vi "DebugProg.vi"() -> ()   [LabVIEW 2009]
panel:
  out "ALG output array":T1(array[cluster])
  out "appended path":path
  out "VOC Input varables type":string[](array[string])
  out "VOC Output varables type":string[](array[string])
  out "VOC Input varables names":string[](array[string])
  out "VOC Output varables names":string[](array[string])
  out "VOC Output varables ports":i32[](array[numeric])
  out "VOC Input varables bytes":i32[](array[numeric])
  out "VOC Output varables bytes":i32[](array[numeric])
  out "VOC Input varables ports":i32[](array[numeric])
  out "Array":u8[](array[numeric])
  out "Result Input FOR VOC":u8[](array[numeric])
  out "ALG MSG  PARAM 2":enum16{"void", "byte", "int", "float"}(ring)
  out "CA Output varables names":string[](array[string])
  out "CA Output varables type":string[](array[string])
  out "AY Input varables names":string[](array[string])
  out "AY Input varables type":string[](array[string])
  out "Output ALG Msg Last Iter":string[][](table)
  out "Output VOC Msg Last Iter":string[][](table)
  out "Curr step ALG msg counter":i32
  out "Curr step VOC MSG counter":i32
  in  "Mode":bool
  in  "stop 2":bool
  in  "run":bool
  in  "Tab Control":T2(tab)
  out "Очередь сообщений для АУ":i32(slide)
  in  "send ALG msg":bool
  in  "Параметр сообщения для АУ":string
  in  "Код сообщения для АУ":string(combo)
  out "Очередь сообщений для  ВОУ":i32(slide)
  in  "send voc msg 2":bool
  in  "Параметр сообщения для ВОУ":string
  in  "Код сообщения для ВОУ":string(combo)
  in  "Тип параметра сообщения для АУ":enum16{"void", "byte", "int", "float"}(ring)
  in  "Тип параметра сообщения для ВОУ":enum16{"void", "byte", "int", "float"}(ring)
  out "Выходные глобальные переменные АУ":string[][](table)
  in  "Входные глобальные переменные АУ":string[][](table)
  in  "Значение порта АУ":u8
  in  "Ручное управление портом АУ":bool
  in  "Установить новое значение порта АУ":bool
  in  "ALG Input Ports":i32(listbox) caption="Входные порты АУ"
  out "Выходные глобальные переменные ВОУ":string[][](table)
  in  "Значение порта ВОУ":u8
  in  "Ручное управление портом ВОУ":bool
  in  "Установить новое значение порта ВОУ":bool
  in  "Входные глобальные переменные ВОУ":string[][](table)
  in  "Входные порты ВОУ":i32(listbox)
  in  "Выходные сообщения от АУ на последнем шаге":i32(listbox)
  out "Отладочная информация процессов АУ":string[][](table)
  out "Список выходных сообщений от АУ":string[][](table)
  in  "Выходные сообщения от ВОУ на последнем шаге":i32(listbox)
  out "Список выходных сообщений от ВОУ":string[][](table)
  out "Отладочная информация процессов ВОУ":string[][](table)
  in  "stop":bool
  # "ПОШАГОВЫЙ РЕЖИМ"
  # "НЕПРЕРЫВНЫЙ РЕЖИМ"
  # "Входные сообщения АУ"
  # "Входные сообщения ВОУ"
  # "Порядок создания нового проекта:\n\n1)\tИз папки \"C:\\ProgramData\\ManualComplexData\" Скопируйте папки CA, VOC и файл cfg.xml в директорию проекта. \n2)\tЗакройте программу ручной отладки, если она была у вас открыта.\n3)\tВ папке CA в файле CA.rcs опишите алгоритм управления. Запустите скрипт ManualBuild.\n4)\tВ папке VOC в файле voc.rcs опишите алгоритм управления. Запустите скрипт ManualBuild."
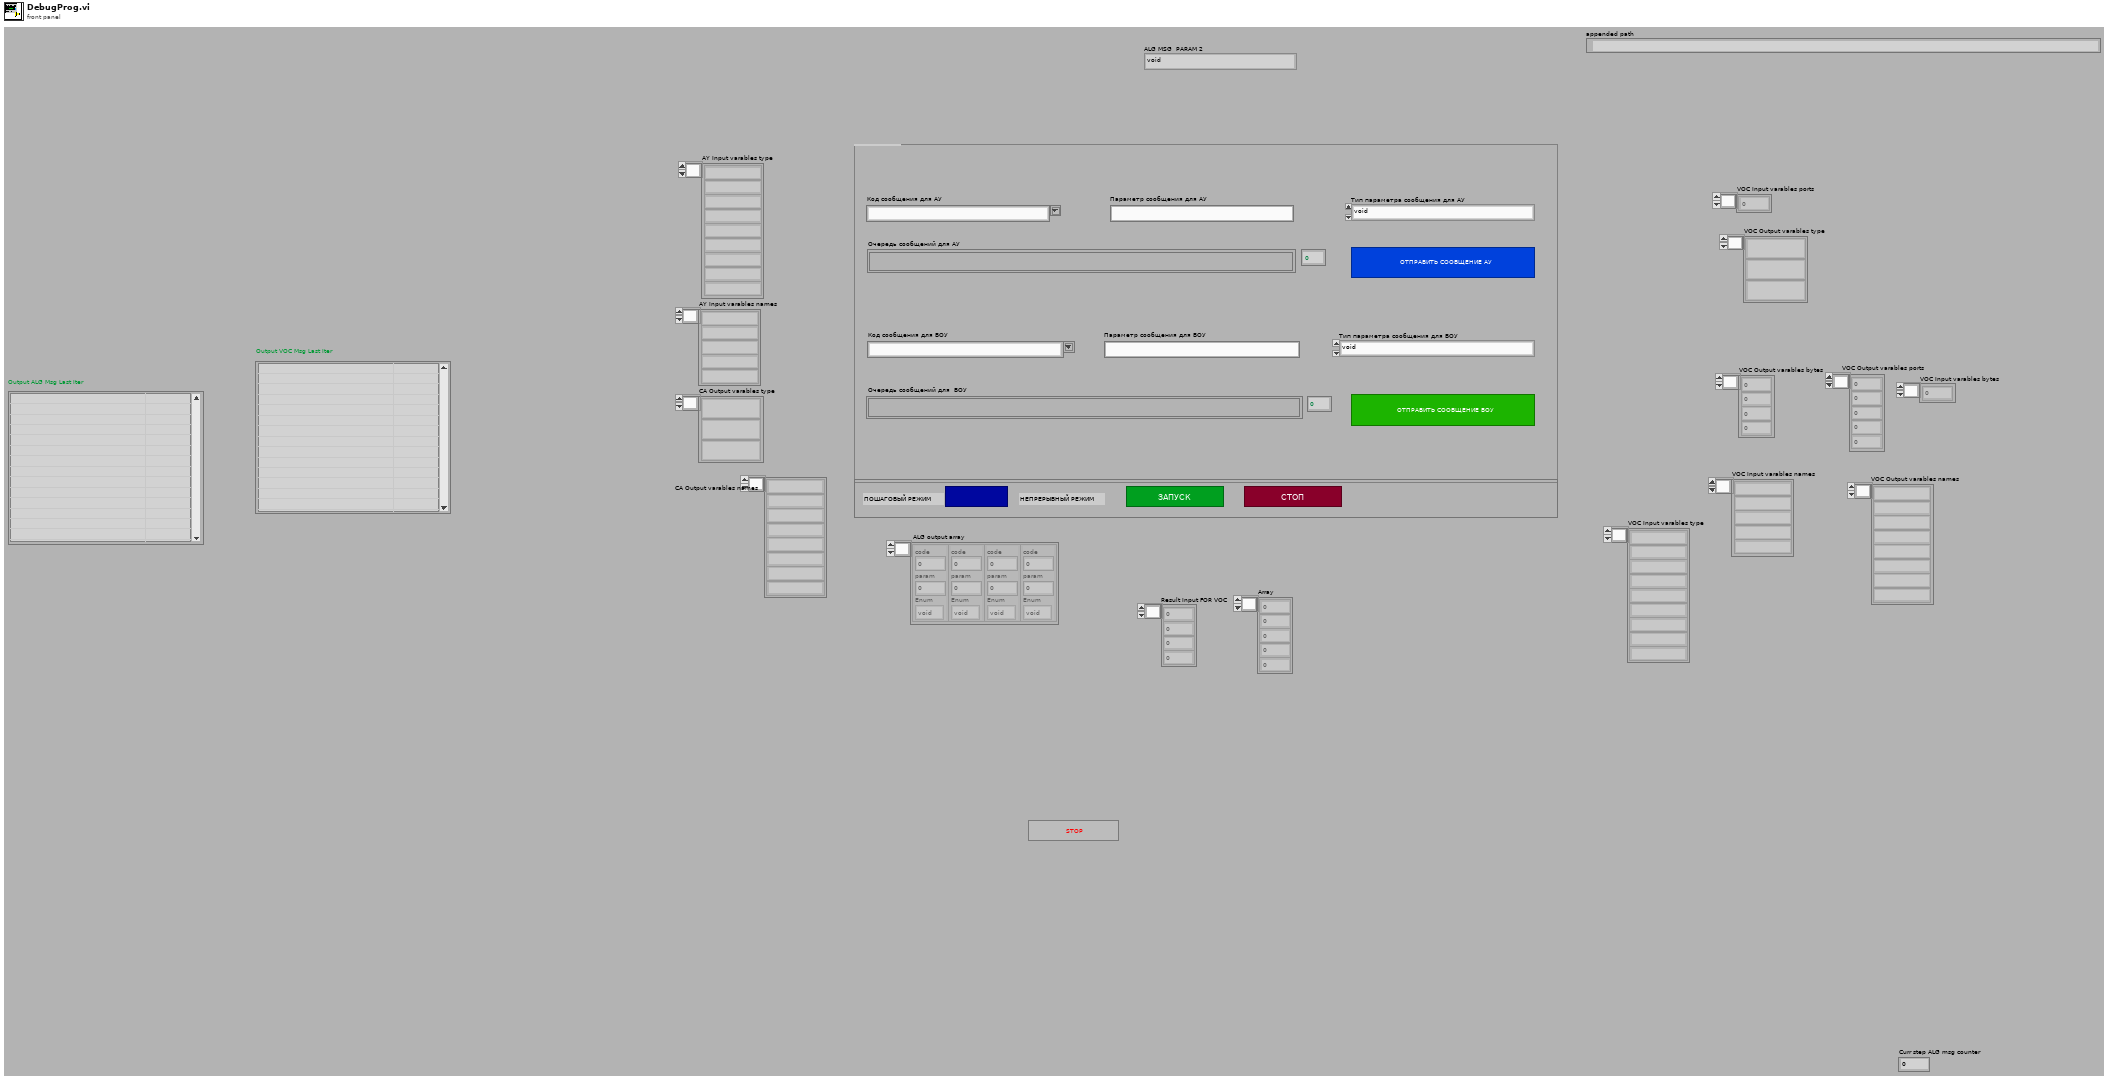
[diagram p1: front panel]
types:
  T1 = cluster{"code":i32, "param":i32, "Enum":enum16{"void", "byte", "int", "float"}}[]
  T2 = enum32{"Генерация входных сообщений АУ и ВОУ", "Переменные АУ", "Переменные ВОУ", "Отладочная информация АУ", "Отладочная информация ВОУ", "Помощь"}
  T3 = enum8{"Enabled", "Disabled", "Disabled and Grayed Out"}
  T4 = cluster{"code":i32, "param":i32, "Enum":enum16{"void", "byte", "int", "float"}}
  T5 = cluster{"trimmed string":string, "trimmed string":string}[]
  T6 = cluster{i32, "Casted Parameter":i32, "Тип параметра сообщения для АУ":enum16{"void", "byte", "int", "float"}}
  T7 = cluster{i32, "Casted Parameter":i32, "Тип параметра сообщения для ВОУ":enum16{"void", "byte", "int", "float"}}
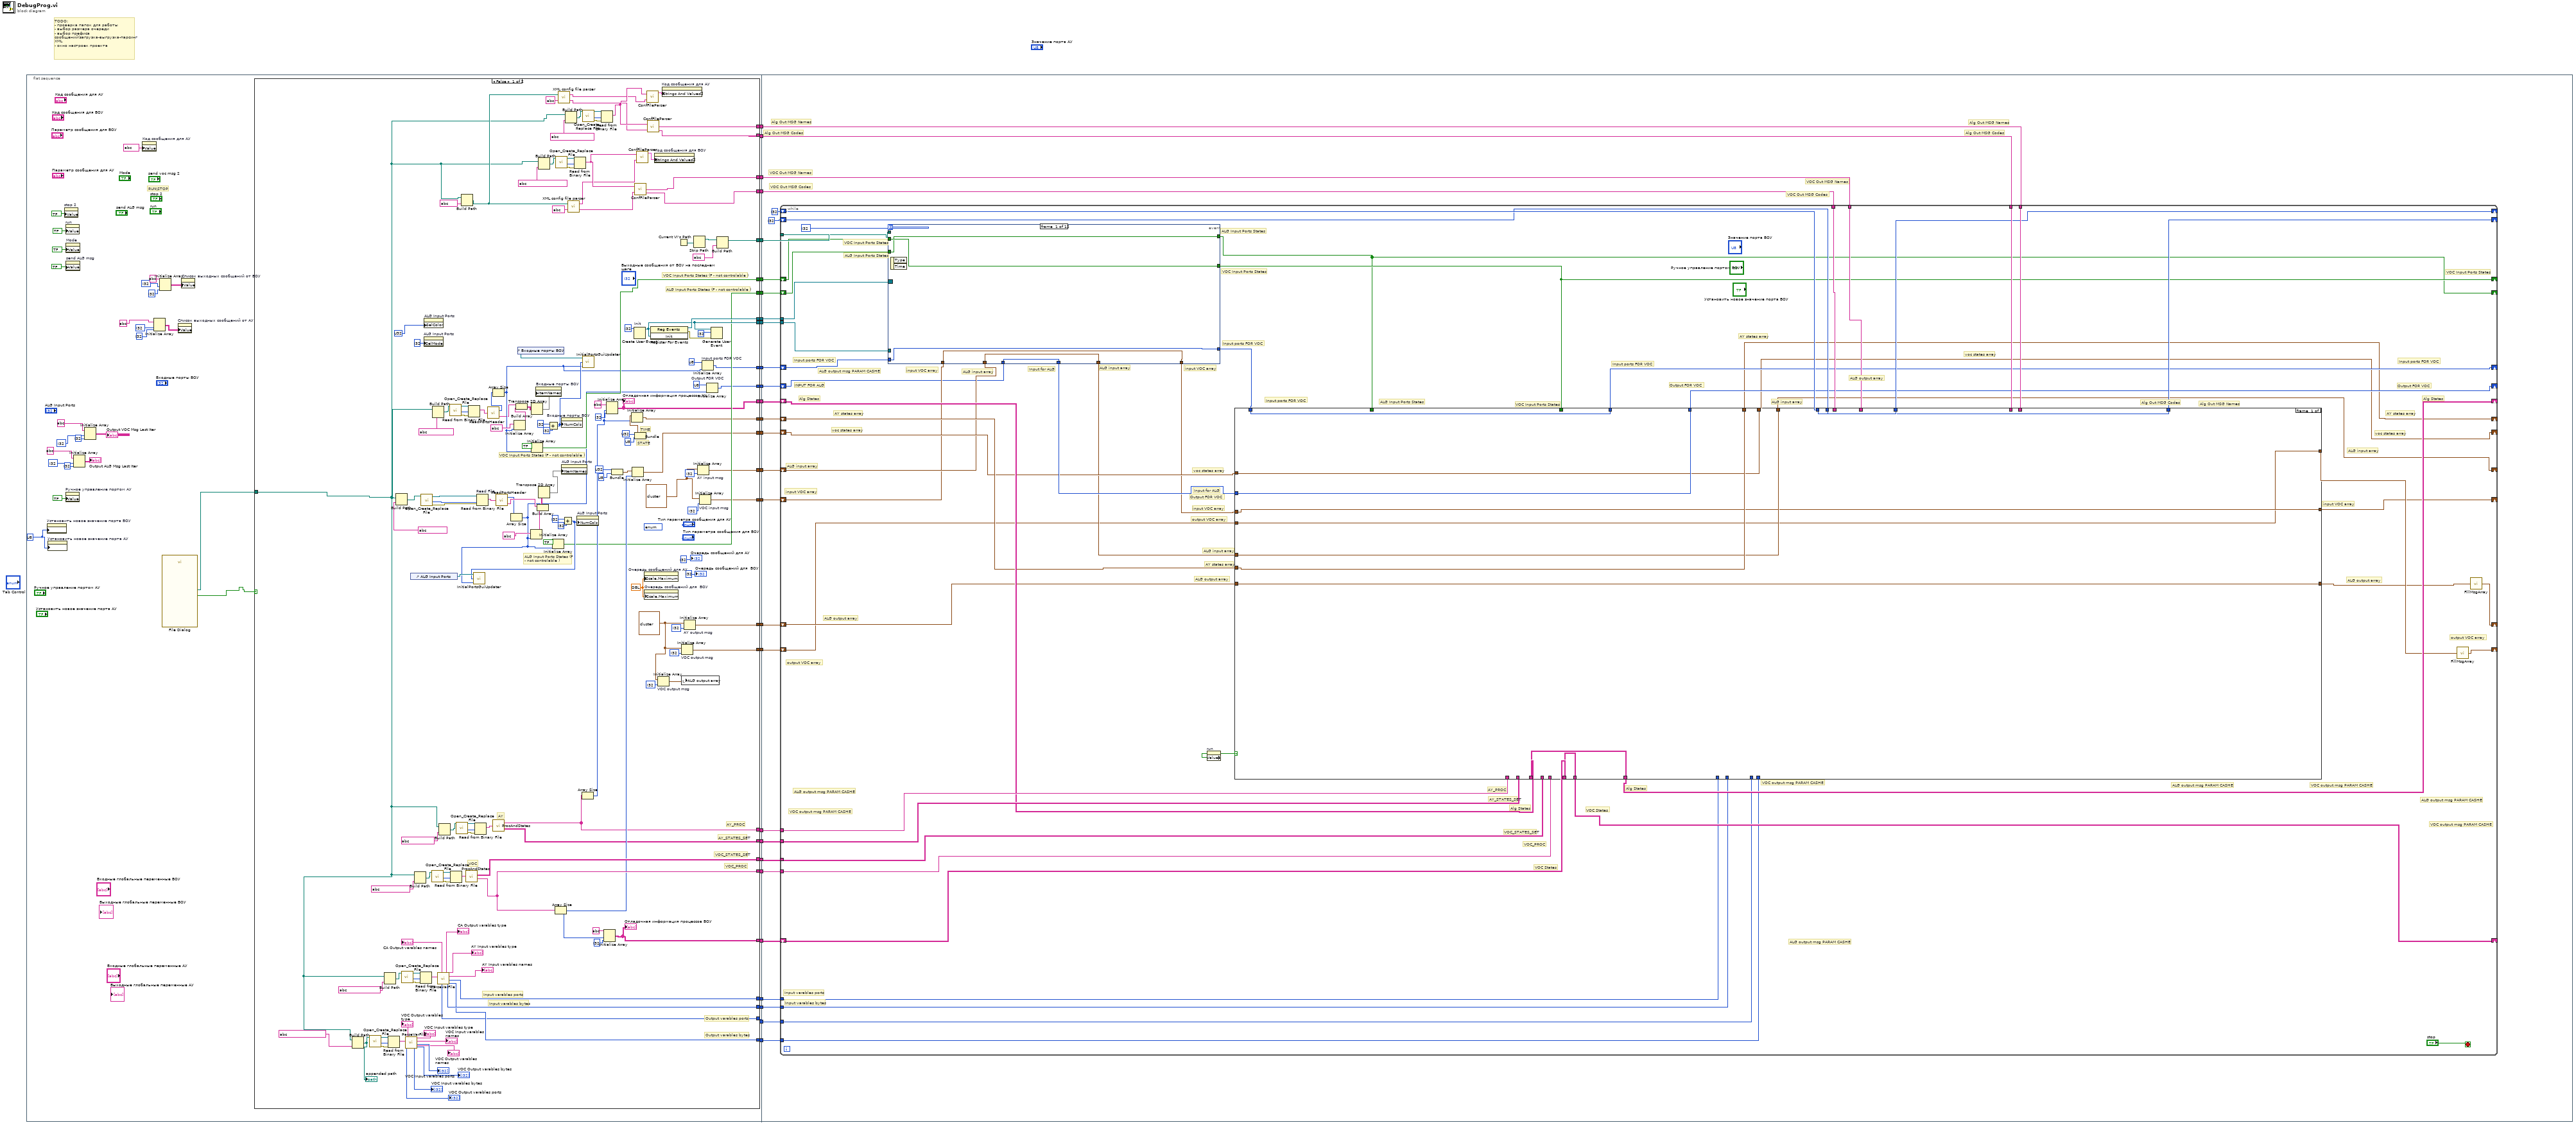
[diagram p0: block diagram]
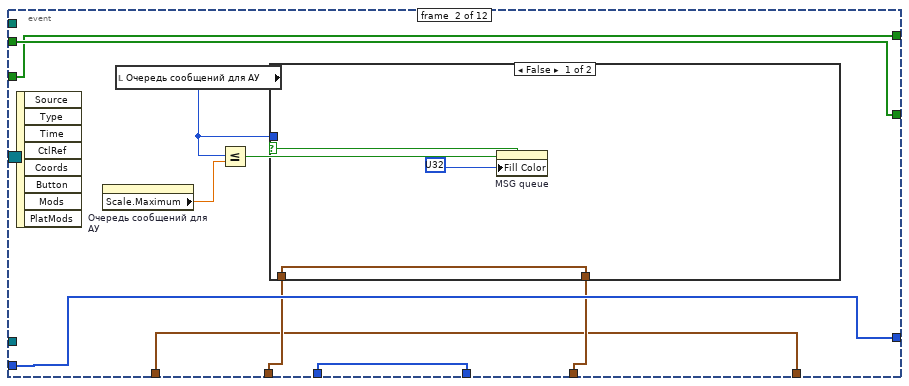
[diagram p3: hidden frame]
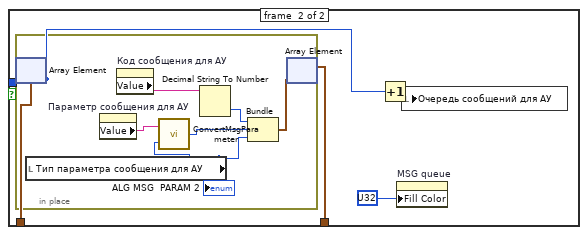
[diagram p4: hidden frame]
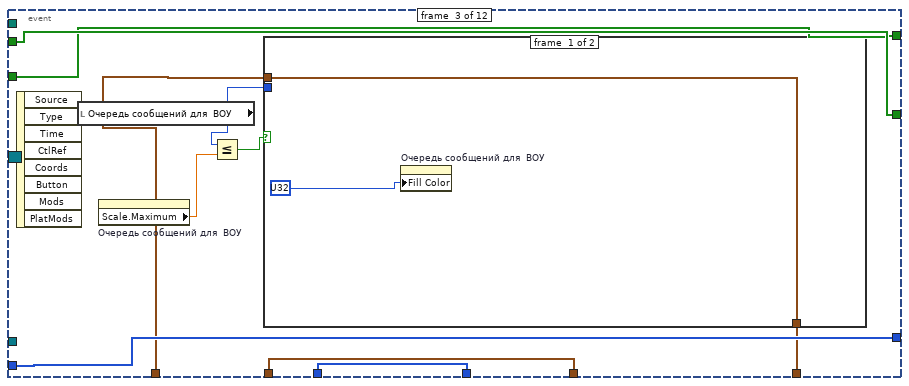
[diagram p5: hidden frame]
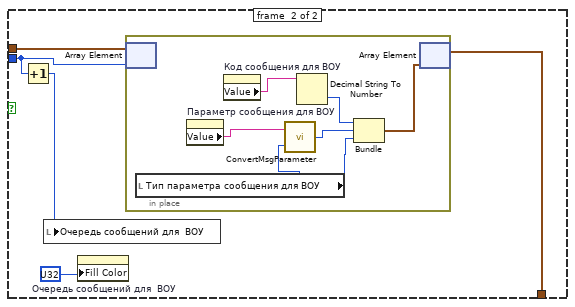
[diagram p6: hidden frame]
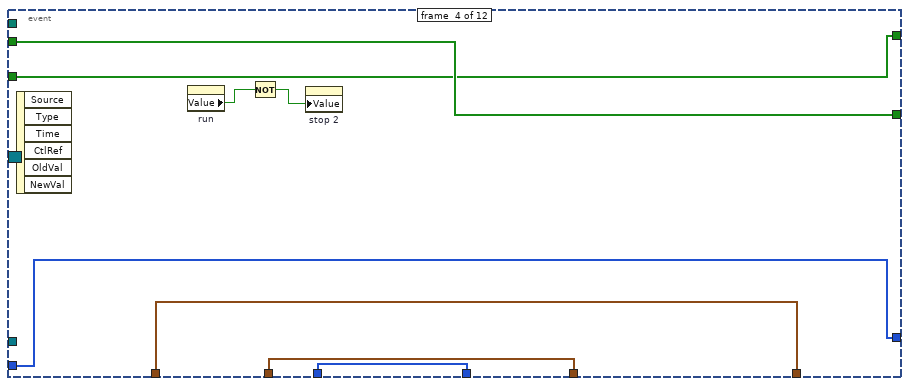
[diagram p7: hidden frame]
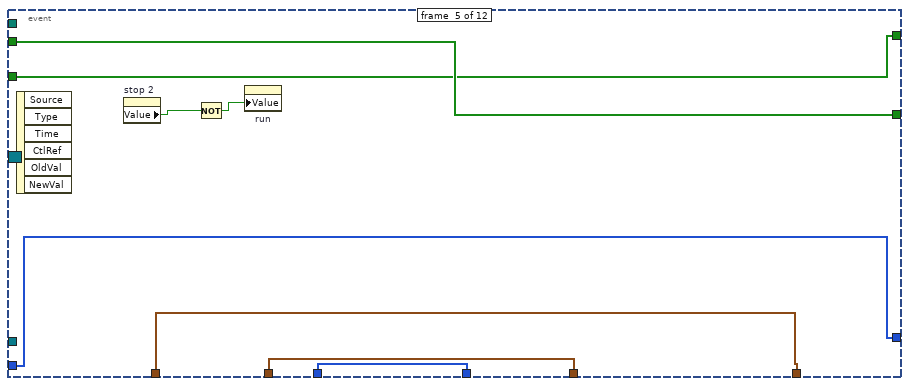
[diagram p8: hidden frame]
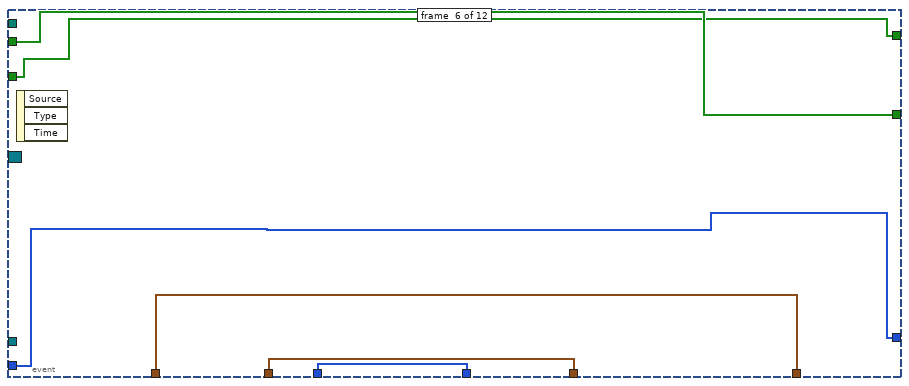
[diagram p9: hidden frame]
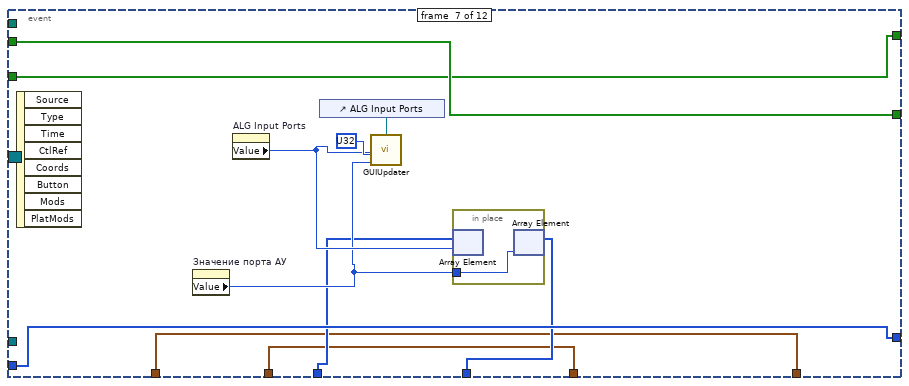
[diagram p10: hidden frame]
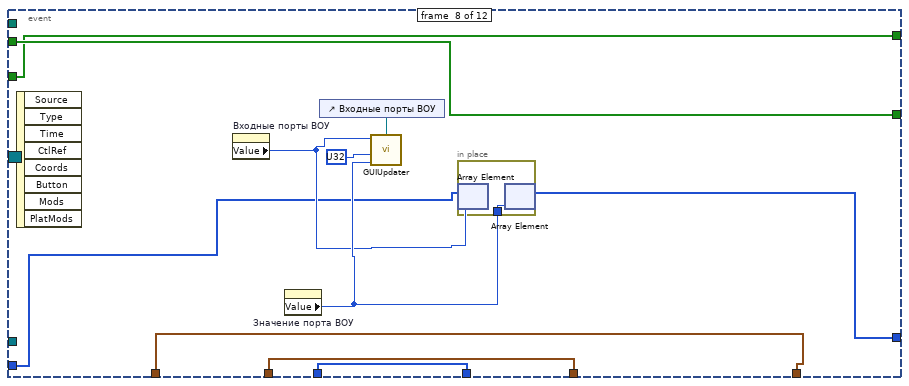
[diagram p11: hidden frame]
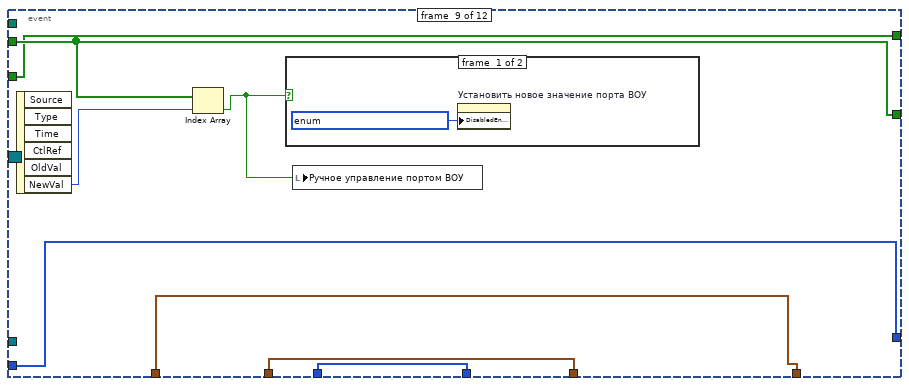
[diagram p12: hidden frame]
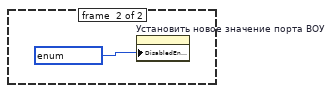
[diagram p13: hidden frame]
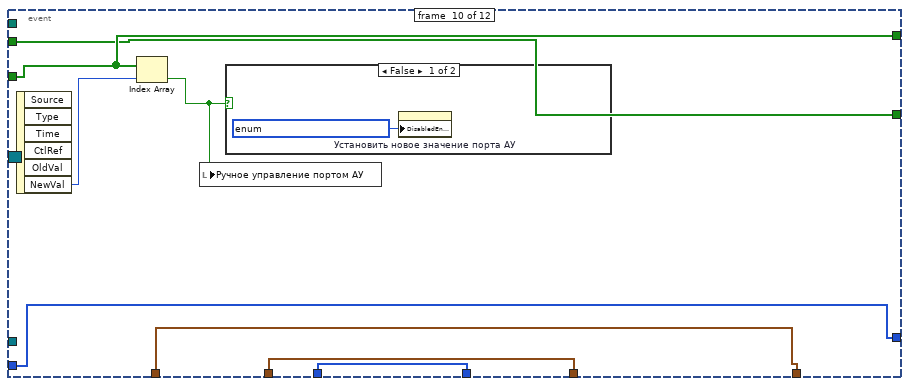
[diagram p14: hidden frame]
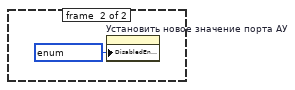
[diagram p15: hidden frame]
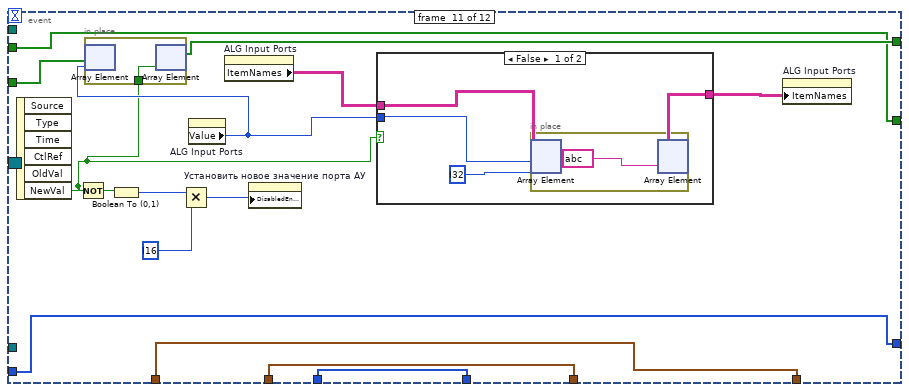
[diagram p16: hidden frame]
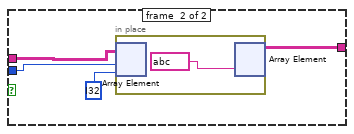
[diagram p17: hidden frame]
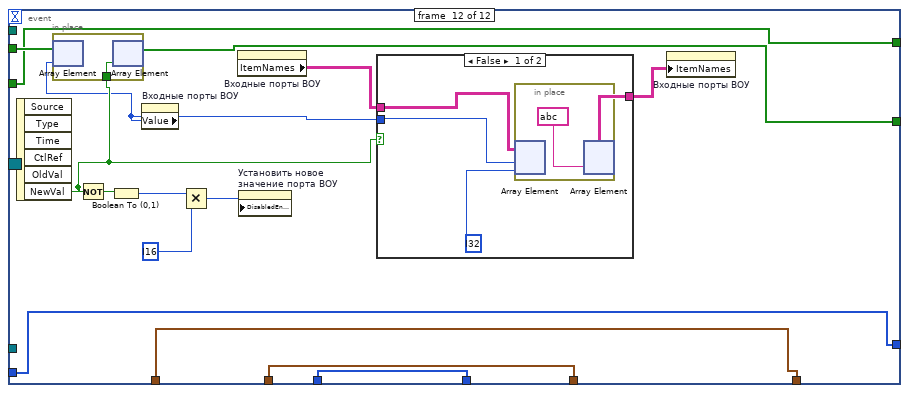
[diagram p18: hidden frame]
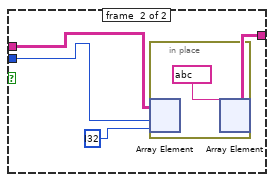
[diagram p19: hidden frame]
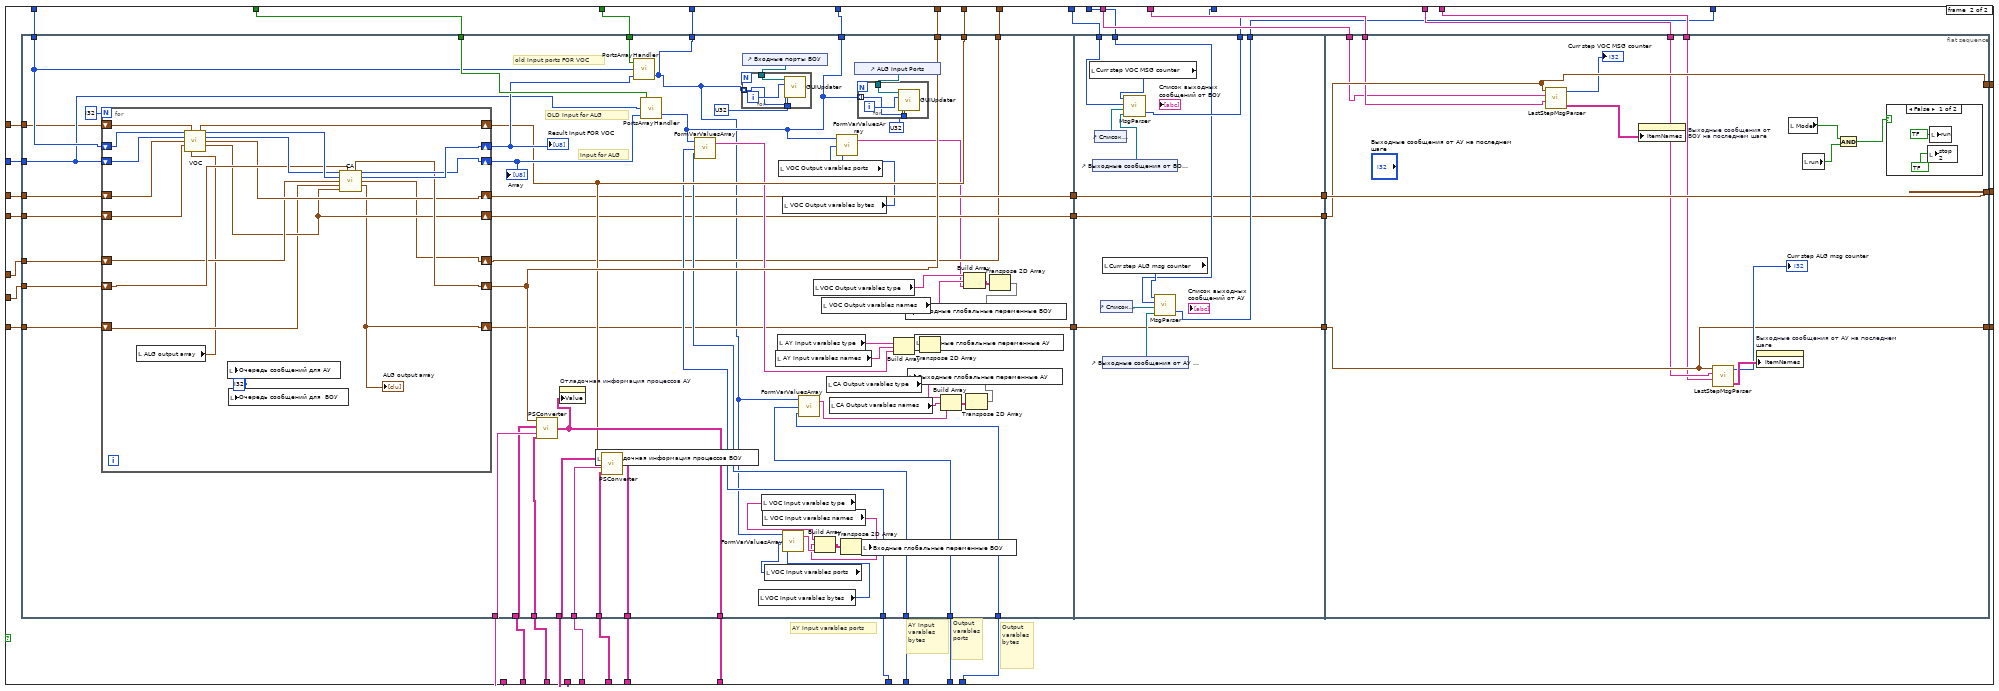
[diagram p20: hidden frame]
diagram:
  # "TODO:\n- проверка папок для работы\n- выбор размера очереди\n- выбор префиса сообщений(загрузка-выгрузка-парсинг XML\n- окно настроек проекта"
  n1 = flat-sequence {
    tunnel: [w74] -> w27
    tunnel: [w72] -> w26
    tunnel: [w73] -> w25
    tunnel: [w71] -> w24
    tunnel: [w70] -> w23
    tunnel: [w69] -> w22
    tunnel: [w68] -> w21
    tunnel: [w47] -> w20
    tunnel: [w46] -> w19
    tunnel: [w58] -> w18
    tunnel: [w61] -> w17
    tunnel: [w45] -> w16
    tunnel: [w44] -> w15
    tunnel: [w43] -> w14
    tunnel: [w42] -> w13
    tunnel: [w41] -> w12
    tunnel: [w40] -> w11
    tunnel: [w39] -> w10
    tunnel: [w38] -> w9
    tunnel: [w37] -> w8
    tunnel: [w36] -> w7
    tunnel: [w35] -> w6
    tunnel: [w34] -> w5
    tunnel: [w31] -> w4
    tunnel: [w33] -> w3
    tunnel: [w30] -> w2
    tunnel: [w32] -> w1
    tunnel: w27 -> [w263]
    tunnel: w26 -> [w262]
    tunnel: w25 -> [w261]
    tunnel: w24 -> [w258]
    tunnel: w23 -> [w257]
    tunnel: w22 -> [w260]
    tunnel: w21 -> [w259]
    tunnel: w20 -> [w255]
    tunnel: w19 -> [w254]
    tunnel: w18 -> [w253]
    tunnel: w17 -> [w252]
    tunnel: w16 -> [w250]
    tunnel: w15 -> [w249]
    tunnel: w14 -> [w248]
    tunnel: w13 -> [w247]
    tunnel: w12 -> [w246]
    tunnel: w11 -> [w245]
    tunnel: w10 -> [w244]
    tunnel: w9 -> [w238]
    tunnel: w8 -> [w237]
    tunnel: w7 -> [w236]
    tunnel: w6 -> [w235]
    tunnel: w5 -> [w243]
    tunnel: w4 -> [w242]
    tunnel: w3 -> [w241]
    tunnel: w2 -> [w240]
    tunnel: w1 -> [w239]
    frame #0 {
      w48 = u8 ? ("Disabled")
      # "RUN\\STOP"
      n2 = property on="Установить новое значение порта ВОУ" class="Bool (strict)"("DisabledEnum"=w48) -> ()  [unwired: 2 in, 2 out]
      n3 = property on="Установить новое значение порта АУ" class="Bool (strict)"("DisabledEnum"=w48) -> ()  [unwired: 2 in, 2 out]
      n4 = property on="stop 2" class="Bool (strict)"("Value"=bool ? ("send msg 3")) -> ()  [unwired: 2 in, 2 out]
      n5 = property on="run" class="Bool (strict)"("Value"=bool ? ("send msg 2")) -> ()  [unwired: 2 in, 2 out]
      n6 = property on="Ручное управление портом АУ" class="Bool (strict)"("Value"=bool ? ("Controlable")) -> ()  [unwired: 2 in, 2 out]
      n7 = property on="Mode" class="Bool (strict)"("Value"=bool ? ("Mode")) -> ()  [unwired: 2 in, 2 out]
      n8 = property on="send ALG msg" class="Bool (strict)"("Value"=bool ? ("send msg")) -> ()  [unwired: 2 in, 2 out]
      n9 = Initialize Array(string ? ("Value"), i32 ? ("dimension size"), i32 ? ("dimension size")) -> (→"Output ALG Msg Last Iter":string[][])
      n10 = Initialize Array(string ? ("Value"), i32 ? ("dimension size"), i32 ? ("dimension size")) -> (→"Output VOC Msg Last Iter":string[][])
      n11 = property on="Код сообщения для АУ" class="CmbBox"("Value"=string ? ("CODE")) -> ()  [unwired: 2 in, 2 out]
      n12 = Initialize Array(string ? ("element"), i32 ? ("dimension size"), i32 ? ("dimension size")) -> (w66:string[][])
      n13 = Initialize Array(string ? ("element"), i32 ? ("dimension size"), i32 ? ("dimension size")) -> (w67:string[][])
      n14 = call "File Dialog"() -> ("selected path"=w29:path, "cancelled"=w28:bool)  [unwired: 12 in, 2 out]
      n15 = property on="Список выходных сообщений от АУ" class="Tbl (strict)"("Value"=w66) -> ()  [unwired: 2 in, 2 out]
      n16 = property on="Список выходных сообщений от ВОУ" class="Tbl (strict)"("Value"=w67) -> ()  [unwired: 2 in, 2 out]
      n17 = case shown="False" w28 {
        tunnel: [w195 _] -> w74
        tunnel: [w191 _] -> w73
        tunnel: [w189 _] -> w72
        tunnel: [w187 _] -> w71
        tunnel: [w186 _] -> w70
        tunnel: [w185 _] -> w69
        tunnel: [w184 _] -> w68
        tunnel: [w178 _] -> w61
        tunnel: [w177 _] -> w58
        tunnel: [w152 _] -> w47
        tunnel: [w151 _] -> w46
        tunnel: [w148 _] -> w45
        tunnel: [w146 _] -> w44
        tunnel: [w143 _] -> w43
        tunnel: [w142 _] -> w42
        tunnel: [w141 _] -> w41
        tunnel: [w140 _] -> w40
        tunnel: [w139 _] -> w39
        tunnel: [w138 _] -> w38
        tunnel: [w137 _] -> w37
        tunnel: [w136 _] -> w36
        tunnel: [w135 _] -> w35
        tunnel: [w134 _] -> w34
        tunnel: [w127 _] -> w33
        tunnel: [w126 _] -> w32
        tunnel: [w119 _] -> w31
        tunnel: [w108 _] -> w30
        tunnel: w29 -> [w83 _]
        frame #0 {
          w107 = dbl ? ("Scale.Range:Maximum")
          (unwired) enum16{"void", "byte", "int", "float"} ? ("Enum")
          w120 = T4 ? ("Cluster")
          w80 = T4 ? ("Cluster")
          w194 = i32 ?  # Init
          # "Output varables bytes"
          # "Output varables ports"
          # "Input varables bytes"
          # "Input varables ports"
          # "VOC Input Ports States (F - not controlable )"
          # "ALG Input Ports States (F - not controlable )"
          # "VOC Input Ports States (F - not controlable )"
          # "ALG Input Ports States (F - not controlable )"
          # "AY"
          # "VOC"
          # "VOC_STATES_SET"
          # "VOC_PROC"
          # "AY_STATES_SET"
          # "AY_PROC"
          # "STATE"
          # "TIME"
          n18 = Build Path(base path=w83, name or relative path=string ?) -> (appended path=w94:path)
          "appended path" <- w94
          n19 = call <vilib>:"Open_Create_Replace File.vi"("file path"=w94) -> ("error out"=w104:errorcluster, "file size (bytes)"=w105:i32, "refnum"=w93:refnum<file>)  [unwired: 7 in, 1 out]
          n20 = Build Path(base path=w83, name or relative path=string ?) -> (appended path=w131:path)
          n21 = Read from Binary File(8:w104, 10:w105, 11:w93) -> (2:w106:string)  [unwired: 3 in, 3 out]
          n22 = Build Path(base path=w83, name or relative path=string ?) -> (appended path=w175:path)
          n23 = call <vilib>:"Open_Create_Replace File.vi"("file path"=w131) -> ("error out"=w133:errorcluster, "file size (bytes)"=w132:i32, "refnum"=w121:refnum<file>)  [unwired: 7 in, 1 out]
          n24 = call "ParseVarFile.vi"("data"=w106) -> ("Output varables bytes"=→"VOC Output varables bytes":i32[], "Output varables names"=→"VOC Output varables names":string[], "Input varables ports"=→"VOC Input varables ports":i32[], "Input varables names"=→"VOC Input varables names":string[], "Output varables type"=→"VOC Output varables type":string[], "Input varables type"=→"VOC Input varables type":string[], "Input varables bytes"=→"VOC Input varables bytes":i32[], "Output varables ports"=→"VOC Output varables ports":i32[])
          n25 = control-ref of="ALG Input Ports"() -> (w157:refnum<vi>)
          n26 = Build Path(base path=w83, name or relative path=string ?) -> (appended path=w214:path)
          n27 = Read from Binary File(8:w133, 10:w132, 11:w121) -> (2:w130:string)  [unwired: 3 in, 3 out]
          n28 = call <vilib>:"Open_Create_Replace File.vi"("file path"=w175) -> ("error out"=w174:errorcluster, "file size (bytes)"=w173:i32, "refnum"=w172:refnum<file>)  [unwired: 7 in, 1 out]
          n29 = property on="ALG Input Ports" class="MCListbox (strict)"("SelMode"=i32 ? ("Selection Mode")) -> ()  [unwired: 2 in, 2 out]
          n30 = property on="ALG Input Ports" class="MCListbox (strict)"("SelColor"=u32 ?) -> ()  [unwired: 2 in, 2 out]
          n31 = call <vilib>:"Open_Create_Replace File.vi"("file path"=w214) -> ("error out"=w213:errorcluster, "file size (bytes)"=w212:i32, "refnum"=w211:refnum<file>)  [unwired: 7 in, 1 out]
          n32 = Build Path(base path=w83, name or relative path=string ?) -> (appended path=w166:path)
          n33 = call "ParseVarFile.vi"("data"=w130) -> ("Output varables bytes"=w126:i32[], "Output varables names"=→"CA Output varables names":string[], "Input varables ports"=w119:i32[], "Input varables names"=→"AY Input varables names":string[], "Output varables type"=→"CA Output varables type":string[], "Input varables type"=→"AY Input varables type":string[], "Input varables bytes"=w127:i32[], "Output varables ports"=w108:i32[])
          n34 = Build Path(base path=w83, name or relative path=string ?) -> (appended path=w208:path)
          n35 = call <vilib>:"Open_Create_Replace File.vi"("file path"=w166) -> ("error out"=w165:errorcluster, "file size (bytes)"=w164:i32, "refnum"=w163:refnum<file>)  [unwired: 7 in, 1 out]
          n36 = Read from Binary File(8:w213, 10:w212, 11:w211) -> (2:w188:string)  [unwired: 3 in, 3 out]
          n37 = call <vilib>:"Open_Create_Replace File.vi"("file path"=w208) -> ("error out"=w207:errorcluster, "file size (bytes)"=w206:i32, "refnum"=w205:refnum<file>)  [unwired: 7 in, 1 out]
          n38 = Build Path(base path=w83, name or relative path=string ?) -> (appended path=w85:path)
          n39 = call "ProcAndStates.vi"("spreadsheet string"=w188) -> ("PROCESSES"=w177:string[], "STATES"=w178:string[][])
          n40 = Read from Binary File(8:w165, 10:w164, 11:w163) -> (2:w118:string)  [unwired: 3 in, 3 out]
          n41 = Read from Binary File(8:w207, 10:w206, 11:w205) -> (2:w216:string)  [unwired: 3 in, 3 out]
          n42 = Read from Binary File "Read File"(8:w174, 10:w173, 11:w172) -> (2:w113:string)  [unwired: 3 in, 3 out]
          n43 = call "ReadPortsHeader.vi"("data"=w118) -> ("Numbers"=w117:i32[], "Names"=w115:string[])
          n44 = Array Size(array=w117) -> (size(s)=w116:i32)
          n45 = call "ProcAndStates.vi"("spreadsheet string"=w216) -> ("PROCESSES"=w152:string[], "STATES"=w151:string[][])
          n46 = call "ReadPortsHeader.vi"("data"=w113) -> ("Numbers"=w110:i32[], "Names"=w112:string[])
          n47 = Array Size(array=w110) -> (size(s)=w109:i32)
          n48 = Initialize Array(string ? ("name or relative path"), w116) -> (w160:string[])
          n49 = Build Array(w115, w160) -> (w159:string[][])
          n50 = control-ref of="Входные порты ВОУ"() -> (w155:refnum<vi>)
          n51 = Initialize Array(string ? ("name or relative path"), w109) -> (w169:string[])
          n52 = Transpose 2D Array(2D array=w159) -> (transposed array=w147:string[][])
          n53 = Initialize Array(bool ? ("Controlable"), w116) -> (w146:bool[])
          n54 = property on="Входные порты ВОУ" class="MCListbox (strict)"("ItemNames"=w147) -> ()  [unwired: 2 in, 2 out]
          n55 = Build Array(w112, w169) -> (w170:string[][])
          n56 = Build Path(base path=w83, name or relative path=string ?) -> (appended path=w229:path)
          n57 = Transpose 2D Array(2D array=w170) -> (transposed array=w168:string[][])
          n58 = Add(x=i32 ?, y=i32 ?) -> (x+y=w154:i32)
          n59 = Initialize Array(bool ? ("Controlable"), w109) -> (w148:bool[])
          n60 = Array Size(array=w177) -> (size(s)=w176:i32)
          n61 = call <vilib>:"Open_Create_Replace File.vi"("file path"=w229) -> ("error out"=w228:errorcluster, "file size (bytes)"=w227:i32, "refnum"=w226:refnum<file>)  [unwired: 7 in, 1 out]
          n62 = call "XML config file parser.vi"("Tag Name"=string ?, "XML File Path"=w85) -> ("Out"=w90:string, "In"=w91:string)
          n63 = property on="Входные порты ВОУ" class="MCListbox (strict)"("NumCols"=w154) -> ()  [unwired: 2 in, 2 out]
          n64 = property on="ALG Input Ports" class="MCListbox (strict)"("ItemNames"=w168) -> ()  [unwired: 2 in, 2 out]
          n65 = Add(x=i32 ?, y=i32 ?) -> (x+y=w156:i32)
          n66 = call "InitialPortsGuiUpdater.vi"("Ports counter"=w109, "port max size"=w156, "MCListbox Refnum"=w157) -> ()
          n67 = Build Path(base path=w83, name or relative path=string ?) -> (appended path=w204:path)
          n68 = call "XML config file parser.vi"("Tag Name"=string ?, "XML File Path"=w85) -> ("Out"=w87:string, "In"=w88:string)
          n69 = Read from Binary File(8:w228, 10:w227, 11:w226) -> (2:w230:string)  [unwired: 3 in, 3 out]
          n70 = property on="ALG Input Ports" class="MCListbox (strict)"("NumCols"=w156) -> ()  [unwired: 2 in, 2 out]
          n71 = Array Size(array=w152) -> (size(s)=w180:i32)
          n72 = call <vilib>:"Open_Create_Replace File.vi"("file path"=w204) -> ("error out"=w203:errorcluster, "file size (bytes)"=w202:i32, "refnum"=w201:refnum<file>)  [unwired: 7 in, 1 out]
          n73 = call "InitialPortsGuiUpdater.vi"("Ports counter"=w116, "port max size"=w154, "MCListbox Refnum"=w155) -> ()
          n74 = Read from Binary File(8:w203, 10:w202, 11:w201) -> (2:w223:string)  [unwired: 3 in, 3 out]
          n75 = Initialize Array(string ? ("Value"), w176, i32 ? ("dimension size")) -> (w134:string[][])
          "Отладочная информация процессов ВОУ" <- w134
          n76 = Initialize Array(string ? ("Value"), w180, i32 ? ("dimension size")) -> (w141:string[][])
          "Отладочная информация процессов АУ" <- w141
          n77 = Bundle(u32 ?, u8 ?) -> (w222:cluster{u32, u8})  [unwired: 1 in]
          n78 = Initialize Array(w222, w176) -> (w139:cluster{u32, u8}[])
          n79 = Create User Event(user event datatype=w194) -> (user event=w189:refnum<user-event>)  [unwired: 1 in, 1 out]
          n80 = call "ConfFileParser.vi"("TEXT"=w230, "search string"=w87) -> ("Names"=w185:string[], "Codes"=w184:string[])  [unwired: 1 out]
          n81 = Bundle(u32 ?, u8 ?) -> (w219:cluster{u32, u8})  [unwired: 1 in]
          n82 = Initialize Array(w219, w180) -> (w140:cluster{u32, u8}[])
          n83 = call "ConfFileParser.vi"("TEXT"=w230, "search string"=w88) -> ("Cluster Array"=w224:T5)  [unwired: 2 out]
          n84 = property on="Очередь сообщений для АУ" class="Slide (strict)"("Scale.Maximum"=w107) -> ()  [unwired: 2 in, 2 out]
          n85 = property on="Очередь сообщений для  ВОУ" class="Slide (strict)"("Scale.Maximum"=w107) -> ()  [unwired: 2 in, 2 out]
          n86 = call "ConfFileParser.vi"("TEXT"=w223, "search string"=w91) -> ("Cluster Array"=w210:T5)  [unwired: 2 out]
          n87 = call "ConfFileParser.vi"("TEXT"=w223, "search string"=w90) -> ("Names"=w187:string[], "Codes"=w186:string[])  [unwired: 1 out]
          n88 = register-events(w189) -> (reference out=w191:refnum<event-registration>, error out=w193:errorcluster)  [unwired: 2 in]
          n89 = property on="Код сообщения для ВОУ" class="CmbBox"("Strings And Values[]"=w224) -> ()  [unwired: 2 in, 2 out]
          n90 = Initialize Array "VOC output msg"(w80, i32 ? ("dimension size")) -> (w81:T1)
          n91 = property on="Код сообщения для АУ" class="CmbBox"("Strings And Values[]"=w210) -> ()  [unwired: 2 in, 2 out]
          n92 = Current VI's Path() -> (path=w197:path)
          n93 = Initialize Array "VOC output msg"(w80, i32 ? ("dimension size")) -> (w135:T1)
          n94 = local write "ALG output array"(w81) -> ()
          n95 = Initialize Array "AY output msg"(w80, i32 ? ("dimension size")) -> (w136:T1)
          n96 = Strip Path(path=w197) -> (stripped path=w196:path)  [unwired: 1 out]
          n97 = Initialize Array "AY input msg"(w120, i32 ? ("dimension size")) -> (w138:T1)
          n98 = Initialize Array "VOC input msg"(w120, i32 ? ("dimension size")) -> (w137:T1)
          n99 = Initialize Array "Input ports FOR VOC"(u8 ? ("element"), w116) -> (w143:u8[])
          n100 = Initialize Array "Output FOR VOC"(u8 ? ("element"), w109) -> (w142:u8[])
          n101 = Generate User Event(user event=w189, event data cluster=i32 ?, error in=w193) -> ()  [unwired: 2 out]
          n102 = Build Path(base path=w196, name or relative path=string ?) -> (appended path=w195:path)
          "Очередь сообщений для  ВОУ" <- i32 ? ("VOC MSG queue")
          "Очередь сообщений для АУ" <- i32 ? ("ALG MSG queue")
        }
        frame #1 {
        }
      }
    }
    frame #1 {
      # "VOC Out MSG Names"
      # "Alg Out MSG Codes"
      # "Alg Out MSG Names"
      # "VOC Out MSG Codes"
      # "VOC Out MSG Codes"
      # "VOC Out MSG Names"
      # "Alg Out MSG Codes"
      # "Alg Out MSG Names"
      n103 = while {
        tunnel: w263 -> [w311]
        tunnel: w262 -> [w313]
        tunnel: w261 -> [w314]
        tunnel: w260 -> [w310]
        tunnel: w259 -> [w309]
        tunnel: w258 -> [w307]
        tunnel: w257 -> [w308]
        shift-right: [w304] -> _
        shift-left: i32 ? -> [w305]
        tunnel: w253 -> [w301]
        tunnel: w255 -> [w303]
        tunnel: w254 -> [w302]
        tunnel: w252 -> [w298]
        shift-right: [w299] -> _
        shift-left: i32 ? -> [w300]
        shift-right: [w295] -> _
        shift-left: w249 -> [w296]
        shift-right: [w294] -> _
        shift-left: w250 -> [w297]
        shift-right: [w291] -> _
        shift-left: w248 -> [w293]
        shift-right: [w289] -> _
        shift-left: w247 -> [w264]
        shift-right: [w287] -> _
        shift-left: w246 -> [w288]
        shift-right: [w285] -> _
        shift-left: w245 -> [w286]
        shift-right: [w283] -> _
        shift-left: w244 -> [w284]
        shift-right: [w280] -> _
        shift-left: w243 -> [w279]
        tunnel: w242 -> [w276]
        tunnel: w241 -> [w275]
        tunnel: w240 -> [w274]
        tunnel: w239 -> [w273]
        shift-right: [w267] -> _
        shift-left: w238 -> [w272]
        shift-right: [w268] -> _
        shift-left: w237 -> [w271]
        shift-right: [w266] -> _
        shift-left: w236 -> [w270]
        shift-right: [w265] -> _
        shift-left: w235 -> [w269]
        stop <- "stop" stop-if-true
        # "Input varables bytes"
        # "Input varables ports"
        # "VOC Input Ports States"
        # "VOC Input Ports States"
        # "VOC Input Ports States"
        # "Input for ALG"
        # "ALG Input Ports States"
        # "ALG Input Ports States"
        # "ALG Input Ports States"
        # "VOC Input Ports States"
        # "Input for ALG"
        # "VOC output msg PARAM CASHE"
        # "VOC output msg PARAM CASHE"
        # "VOC output msg PARAM CASHE"
        # "VOC output msg PARAM CASHE"
        # "ALG output msg PARAM CASHE"
        # "ALG output msg PARAM CASHE"
        # "ALG output msg PARAM CASHE"
        # "ALG output msg PARAM CASHE"
        # "ALG output msg PARAM CASHE"
        # "voc states array"
        # "VOC States"
        # "Alg States"
        # "VOC States"
        # "Alg States"
        # "Alg States"
        # "Alg States"
        # "VOC_STATES_SET"
        # "VOC_PROC"
        # "AY_STATES_SET"
        # "AY_PROC"
        # "AY states array"
        # "ALG output array"
        # "ALG input array"
        # "output VOC array"
        # "ALG output array"
        # "input VOC array"
        # "ALG input array"
        # "voc states array"
        # "AY states array"
        # "Output FOR VOC"
        # "Input ports FOR VOC"
        # "Output FOR VOC"
        # "Input ports FOR VOC"
        # "Alg Out MSG Codes"
        # "Alg Out MSG Names"
        # "ALG output array"
        # "output VOC array"
        # "output VOC array"
        # "ALG output array"
        # "AY states array"
        # "voc states array"
        # "voc states array"
        # "AY states array"
        # "ALG input array"
        # "Output FOR VOC"
        # "INPUT FOR ALG"
        # "input VOC array"
        # "Input ports FOR VOC"
        # "input VOC array"
        # "ALG input array"
        # "input VOC array"
        # "input VOC array"
        # "Input ports FOR VOC"
        # "Input ports FOR VOC"
        # "ALG input array"
        # "ALG input array"
        n104 = event shown="[2] \"send voc msg 2\": Mouse Down" {
          selector: w314 -> [_ _ _ _ _ _ _ _ _ _ _ _]
          dyn-events: _ -> [_ _ _ _ _ _ _ _ _ _ _ _]
          timeout: i32 ? -> [_ _ _ _ _ _ _ _ _ _ _ _]
          tunnel: w313 -> [_ _ _ _ _ _ _ _ _ _ _ _]
          tunnel: w311 -> [_ _ _ _ _ _ _ _ _ _ _ _]
          tunnel: w297 -> [w320 w329 w352 w372 w380 w388 w395 w407 w418 w429 w439 w464]
          tunnel: [w320 w329 w352 w372 w380 w388 w395 w407 w418 w429 w440 w464] -> w294
          tunnel: w296 -> [w321 w330 w353 w373 w381 w389 w396 w408 w419 w428 w438 w468]
          tunnel: [w321 w330 w353 w373 w381 w389 w396 w408 w419 w428 w438 w465] -> w295
          tunnel: w293 -> [w319 w327 w350 w371 w379 w384 w394 w406 w417 w427 w437 w463]
          tunnel: [w319 w327 w350 w371 w379 w384 w394 w405 w417 w427 w437 w463] -> w292
          tunnel: w264 -> [w318 w326 w349 w370 w378 w387 w393 w404 w416 w426 w436 w462]
          tunnel: [w318 w326 w349 w370 w378 w387 w392 w404 w416 w426 w436 w462] -> w290
          tunnel: w272 -> [w317 w325 w348 w369 w377 w386 w391 w403 w415 w425 w435 w461]
          tunnel: [w317 w324 w348 w369 w377 w386 w391 w403 w415 w425 w435 w461] -> w282
          tunnel: w271 -> [w316 w323 w347 w368 w376 w385 w390 w402 w414 w424 w434 w460]
          tunnel: [w316 w323 w346 w368 w376 w385 w390 w402 w414 w424 w434 w460] -> w281
          event #0 {
            n105 = event-data() -> ()  [unwired: 1 in, 2 out]
          }
          event #1 {
            n106 = event-data() -> ()  [unwired: 1 in, 8 out]
            n107 = property on="Очередь сообщений для АУ" class="Slide (strict)"() -> ("Scale.Maximum"=w322:dbl)  [unwired: 2 in, 2 out]
            n108 = local read "Очередь сообщений для АУ"() -> (w328:i32)
            n109 = Less Or Equal?(x=w328, y=w322) -> (x <= y?=w331:bool)
            n110 = case shown="False" w331 {
              tunnel: w328 -> [_ w337]
              tunnel: w325 -> [w332 w335]
              tunnel: [w332 w334] -> w324
              frame #0 {
                n111 = property on="MSG queue" class="Slide (strict)"("Fill Color"=u32 ?) -> ()  [unwired: 2 in, 2 out]
              }
              frame #1 {
                n112 = in-place {
                  n113 = in-place-array #1(w335, w337) -> ()  [unwired: 1 out]
                  n114 = local read "Тип параметра сообщения для АУ"() -> (w341:enum16{"void", "byte", "int", "float"})
                  "ALG MSG  PARAM 2" <- w341
                  n115 = property on="Параметр сообщения для АУ" class="Str"() -> ("Value"=w342:string)  [unwired: 2 in, 2 out]
                  n116 = property on="Код сообщения для АУ" class="CmbBox"() -> ("Value"=w343:string)  [unwired: 2 in, 2 out]
                  n117 = call "ConvertMsgParameter.vi"("MSG  Type"=w341, "MSG  PARAM"=w342) -> ("Casted Parameter"=w340:i32)
                  n118 = Decimal String To Number(string=w343) -> (number=w344:i32)  [unwired: 2 in, 1 out]
                  n119 = Bundle(w344, "Casted Parameter"=w340, "Тип параметра сообщения для АУ"=w341) -> (w339:T6)  [unwired: 1 in]
                  n120 = in-place-array #1(w339) -> (w334:T1)  [unwired: 1 out]
                }
                n121 = Increment(x=w337) -> (x+1=w336:i32)
                n122 = property on="MSG queue" class="Slide (strict)"("Fill Color"=u32 ?) -> ()  [unwired: 2 in, 2 out]
                n123 = local write "Очередь сообщений для АУ"(w336) -> ()
              }
            }
          }
          event #2 {
            n124 = event-data() -> ()  [unwired: 1 in, 8 out]
            n125 = local read "Очередь сообщений для  ВОУ"() -> (w351:i32)
            n126 = property on="Очередь сообщений для  ВОУ" class="Slide (strict)"() -> ("Scale.Maximum"=w345:dbl)  [unwired: 2 in, 2 out]
            n127 = Less Or Equal?(x=w351, y=w345) -> (x <= y?=w354:bool)
            n128 = case shown="True" w354 {
              tunnel: w351 -> [_ w360]
              tunnel: w347 -> [w355 w358]
              tunnel: [w355 w357] -> w346
              frame #0 {
                n129 = property on="Очередь сообщений для  ВОУ" class="Slide (strict)"("Fill Color"=u32 ?) -> ()  [unwired: 2 in, 2 out]
              }
              frame #1 {
                n130 = Increment(x=w360) -> (x+1=w359:i32)
                n131 = local write "Очередь сообщений для  ВОУ"(w359) -> ()
                n132 = property on="Очередь сообщений для  ВОУ" class="Slide (strict)"("Fill Color"=u32 ?) -> ()  [unwired: 2 in, 2 out]
                n133 = in-place {
                  n134 = in-place-array #2(w358, w360) -> ()  [unwired: 1 out]
                  n135 = local read "Тип параметра сообщения для ВОУ"() -> (w363:enum16{"void", "byte", "int", "float"})
                  n136 = property on="Параметр сообщения для ВОУ" class="Str"() -> ("Value"=w364:string)  [unwired: 2 in, 2 out]
                  n137 = property on="Код сообщения для ВОУ" class="CmbBox"() -> ("Value"=w366:string)  [unwired: 2 in, 2 out]
                  n138 = call "ConvertMsgParameter.vi"("MSG  Type"=w363, "MSG  PARAM"=w364) -> ("Casted Parameter"=w362:i32)
                  n139 = Decimal String To Number(string=w366) -> (number=w367:i32)  [unwired: 2 in, 1 out]
                  n140 = Bundle(w367, "Casted Parameter"=w362, "Тип параметра сообщения для ВОУ"=w363) -> (w365:T7)  [unwired: 1 in]
                  n141 = in-place-array #2(w365) -> (w357:T1)  [unwired: 1 out]
                }
              }
            }
          }
          event #3 {
            n142 = event-data() -> ()  [unwired: 1 in, 6 out]
            n143 = property on="run" class="Bool (strict)"() -> ("Value"=w375:bool)  [unwired: 2 in, 2 out]
            n144 = Not(x=w375) -> (.not. x?=w374:bool)
            n145 = property on="stop 2" class="Bool (strict)"("Value"=w374) -> ()  [unwired: 2 in, 2 out]
          }
          event #4 {
            n146 = event-data() -> ()  [unwired: 1 in, 6 out]
            n147 = property on="stop 2" class="Bool (strict)"() -> ("Value"=w383:bool)  [unwired: 2 in, 2 out]
            n148 = Not(x=w383) -> (.not. x?=w382:bool)
            n149 = property on="run" class="Bool (strict)"("Value"=w382) -> ()  [unwired: 2 in, 2 out]
          }
          event #5 {
            n150 = event-data() -> ()  [unwired: 1 in, 3 out]
          }
          event #6 {
            n151 = event-data() -> ()  [unwired: 1 in, 8 out]
            n152 = property on="Значение порта АУ" class="DigNum (strict)"() -> ("Value"=w397:u8)  [unwired: 2 in, 2 out]
            n153 = property on="ALG Input Ports" class="MCListbox (strict)"() -> ("Value"=w398:i32)  [unwired: 2 in, 2 out]
            n154 = control-ref of="ALG Input Ports"() -> (w400:refnum<vi>)
            n155 = call "GUIUpdater.vi"("value"=w397, "Color"=u32 ?, "line"=w398, "MCListbox Refnum"=w400) -> ()
            n156 = in-place {
              in-place-border: w397 -> [w401]
              n157 = in-place-array #3(w393, w398) -> ()  [unwired: 1 out]
              n158 = in-place-array #3(w401) -> (w392:u8[])  [unwired: 1 out]
            }
          }
          event #7 {
            n159 = event-data() -> ()  [unwired: 1 in, 8 out]
            n160 = property on="Входные порты ВОУ" class="MCListbox (strict)"() -> ("Value"=w409:i32)  [unwired: 2 in, 2 out]
            n161 = property on="Значение порта ВОУ" class="DigNum (strict)"() -> ("Value"=w410:u8)  [unwired: 2 in, 2 out]
            n162 = control-ref of="Входные порты ВОУ"() -> (w412:refnum<vi>)
            n163 = call "GUIUpdater.vi"("value"=w410, "Color"=u32 ?, "line"=w409, "MCListbox Refnum"=w412) -> ()
            n164 = in-place {
              in-place-border: w410 -> [w413]
              n165 = in-place-array #4(w406, w409) -> ()  [unwired: 1 out]
              n166 = in-place-array #4(w413) -> (w405:u8[])  [unwired: 1 out]
            }
          }
          event #8 {
            n167 = event-data() -> ("NewVal"=w421:i32)  [unwired: 1 in, 5 out]
            n168 = Index Array(array=w419, index=w421) -> (element=w420:bool)
            n169 = case shown="True" w420 {
              frame #0 {
                n170 = property on="Установить новое значение порта ВОУ" class="Bool (strict)"("DisabledEnum"=T3 ? ("Disabled")) -> ()  [unwired: 2 in, 2 out]
              }
              frame #1 {
                n171 = property on="Установить новое значение порта ВОУ" class="Bool (strict)"("DisabledEnum"=T3 ? ("Disabled")) -> ()  [unwired: 2 in, 2 out]
              }
            }
            n172 = local write "Ручное управление портом ВОУ"(w420) -> ()
          }
          event #9 {
            n173 = event-data() -> ("NewVal"=w431:i32)  [unwired: 1 in, 5 out]
            n174 = Index Array(array=w429, index=w431) -> (element=w430:bool)
            n175 = local write "Ручное управление портом АУ"(w430) -> ()
            n176 = case shown="False" w430 {
              frame #0 {
                n177 = property on="Установить новое значение порта АУ" class="Bool (strict)"("DisabledEnum"=T3 ? ("Disabled")) -> ()  [unwired: 2 in, 2 out]
              }
              frame #1 {
                n178 = property on="Установить новое значение порта АУ" class="Bool (strict)"("DisabledEnum"=T3 ? ("Disabled")) -> ()  [unwired: 2 in, 2 out]
              }
            }
          }
          event #10 {
            n179 = event-data() -> ("NewVal"=w441:bool)  [unwired: 1 in, 5 out]
            n180 = Not(x=w441) -> (.not. x?=w444:bool)
            n181 = Boolean To (0,1)(Boolean=w444) -> (0, 1=w447:i16)
            n182 = Multiply(x=w447, y=i16 ?) -> (x*y=w445:i16)
            n183 = property on="ALG Input Ports" class="MCListbox (strict)"() -> ("Value"=w442:i32)  [unwired: 2 in, 2 out]
            n184 = in-place {
              in-place-border: w441 -> [w449]
              n185 = in-place-array #5(w439, w442) -> ()  [unwired: 1 out]
              n186 = in-place-array #5(w449) -> (w440:bool[])  [unwired: 1 out]
            }
            n187 = property on="ALG Input Ports" class="MCListbox (strict)"() -> ("ItemNames"=w443:string[][])  [unwired: 2 in, 2 out]
            n188 = property on="Установить новое значение порта АУ" class="Bool (strict)"("DisabledEnum"=w445) -> ()  [unwired: 2 in, 2 out]
            n189 = case shown="False" w441 {
              tunnel: w442 -> [w451 w456]
              tunnel: w443 -> [w450 w457]
              tunnel: [w452 w455] -> w448
              frame #0 {
                n190 = in-place {
                  n191 = in-place-array #6(w450, w451, i32 ? ("disabled index (col)")) -> ()  [unwired: 1 out]
                  n192 = in-place-array #6(string ?) -> (w452:string[][])  [unwired: 2 out]
                }
              }
              frame #1 {
                n193 = in-place {
                  n194 = in-place-array #7(w457, w456, i32 ? ("disabled index (col)")) -> ()  [unwired: 1 out]
                  n195 = in-place-array #7(string ?) -> (w455:string[][])  [unwired: 2 out]
                }
              }
            }
            n196 = property on="ALG Input Ports" class="MCListbox (strict)"("ItemNames"=w448) -> ()  [unwired: 2 in, 2 out]
          }
          event #11 {
            n197 = event-data() -> ("NewVal"=w467:bool)  [unwired: 1 in, 5 out]
            n198 = Not(x=w467) -> (.not. x?=w470:bool)
            n199 = Boolean To (0,1)(Boolean=w470) -> (0, 1=w473:i16)
            n200 = property on="Входные порты ВОУ" class="MCListbox (strict)"() -> ("Value"=w466:i32)  [unwired: 2 in, 2 out]
            n201 = in-place {
              in-place-border: w467 -> [w475]
              n202 = in-place-array #8(w468, w466) -> ()  [unwired: 1 out]
              n203 = in-place-array #8(w475) -> (w465:bool[])  [unwired: 1 out]
            }
            n204 = Multiply(x=w473, y=i16 ?) -> (x*y=w471:i16)
            n205 = property on="Входные порты ВОУ" class="MCListbox (strict)"() -> ("ItemNames"=w469:string[][])  [unwired: 2 in, 2 out]
            n206 = property on="Установить новое значение порта ВОУ" class="Bool (strict)"("DisabledEnum"=w471) -> ()  [unwired: 2 in, 2 out]
            n207 = case shown="False" w467 {
              tunnel: w466 -> [w478 w483]
              tunnel: w469 -> [w477 w484]
              tunnel: [w476 w481] -> w474
              frame #0 {
                n208 = in-place {
                  n209 = in-place-array #9(w477, w478, i32 ? ("disabled index (col)")) -> ()  [unwired: 1 out]
                  n210 = in-place-array #9(string ?) -> (w476:string[][])  [unwired: 2 out]
                }
              }
              frame #1 {
                n211 = in-place {
                  n212 = in-place-array #10(w484, w483, i32 ? ("disabled index (col)")) -> ()  [unwired: 1 out]
                  n213 = in-place-array #10(string ?) -> (w481:string[][])  [unwired: 2 out]
                }
              }
            }
            n214 = property on="Входные порты ВОУ" class="MCListbox (strict)"("ItemNames"=w474) -> ()  [unwired: 2 in, 2 out]
          }
        }
        n215 = property on="run" class="Bool (strict)"() -> ("Value"=w306:bool)  [unwired: 2 in, 2 out]
        n216 = case shown="True" w306 {
          tunnel: w310 -> [_ w541]
          tunnel: w309 -> [_ w540]
          tunnel: w308 -> [_ w539]
          tunnel: w307 -> [_ w538]
          tunnel: w305 -> [w497 w533]
          tunnel: [w497 w532] -> w304
          tunnel: w303 -> [_ w537]
          tunnel: w302 -> [_ w536]
          tunnel: w301 -> [_ w535]
          tunnel: w298 -> [_ w534]
          tunnel: w300 -> [w496 w531]
          tunnel: [w496 w530] -> w299
          tunnel: w294 -> [_ w529]
          tunnel: w295 -> [_ w528]
          tunnel: w292 -> [w495 w527]
          tunnel: [w495 w526] -> w291
          tunnel: w290 -> [w494 w525]
          tunnel: [w494 w524] -> w289
          tunnel: w288 -> [w486 w523]
          tunnel: [w486 w522] -> w287
          tunnel: w286 -> [w493 w521]
          tunnel: [w493 w520] -> w285
          tunnel: w284 -> [w492 w519]
          tunnel: [w492 w518] -> w283
          tunnel: w282 -> [w491 w517]
          tunnel: [w491 w516] -> w267
          tunnel: w281 -> [w490 w515]
          tunnel: [w490 w512] -> w268
          tunnel: w270 -> [w489 w511]
          tunnel: [w489 w508] -> w277
          tunnel: w269 -> [w488 w507]
          tunnel: [w488 w504] -> w278
          tunnel: w279 -> [w487 w503]
          tunnel: [w487 w502] -> w280
          tunnel: w276 -> [_ w501]
          tunnel: w275 -> [_ w500]
          tunnel: w274 -> [_ w499]
          tunnel: w273 -> [_ w498]
          frame #0 {
          }
          frame #1 {
            # "Output varables bytes"
            # "Output varables ports"
            # "AY Input varables bytes"
            # "AY Input varables ports"
            n217 = flat-sequence {
              tunnel: w537 -> [w602]
              tunnel: w536 -> [w599]
              tunnel: w535 -> [w601]
              tunnel: w534 -> [w600]
              tunnel: w529 -> [w594]
              tunnel: w528 -> [w593]
              tunnel: w527 -> [w591]
              tunnel: [w556] -> w526
              tunnel: w525 -> [w589]
              tunnel: [w557] -> w524
              tunnel: w523 -> [w587]
              tunnel: [w585] -> w522
              tunnel: w521 -> [w586]
              tunnel: [w584] -> w520
              tunnel: w519 -> [w583]
              tunnel: [w582] -> w518
              tunnel: w517 -> [w563]
              tunnel: [w559] -> w516
              tunnel: w515 -> [w565]
              tunnel: [w561] -> w514
              tunnel: w511 -> [w562]
              tunnel: [w558] -> w510
              tunnel: w507 -> [w564]
              tunnel: [w560] -> w506
              tunnel: w503 -> [w581]
              tunnel: [w580] -> w502
              tunnel: w501 -> [w579]
              tunnel: w500 -> [w578]
              tunnel: w499 -> [w572]
              tunnel: w498 -> [w571]
              tunnel: w533 -> [w642]
              tunnel: [w641] -> w532
              tunnel: w531 -> [w638]
              tunnel: [w639] -> w530
              tunnel: w514 -> [w633]
              tunnel: [w633] -> w513
              tunnel: w510 -> [w632]
              tunnel: [w632] -> w509
              tunnel: w506 -> [w631]
              tunnel: [w631] -> w505
              tunnel: w541 -> [w647]
              tunnel: w540 -> [w646]
              tunnel: w539 -> [w645]
              tunnel: w538 -> [w644]
              tunnel: w513 -> [w657]
              tunnel: [w657] -> w512
              tunnel: w509 -> [w651]
              tunnel: [w651] -> w508
              tunnel: w505 -> [w656]
              tunnel: [w656] -> w504
              frame #0 {
                # "OLD Input for ALG"
                # "Input for ALG"
                # "old Input ports FOR VOC"
                n218 = for {
                  N: i32 ? -> [_]
                  shift-right: [w627] -> w590
                  shift-left: w591 -> [w628]
                  shift-right: [w626] -> w588
                  shift-left: w589 -> [w621]
                  shift-right: [w624] -> w584
                  shift-left: w586 -> [w625]
                  shift-right: [w622] -> w582
                  shift-left: w583 -> [w623]
                  shift-right: [w618] -> w561
                  shift-left: w565 -> [w620]
                  shift-right: [w616] -> w560
                  shift-left: w564 -> [w619]
                  shift-right: [w614] -> w559
                  shift-left: w563 -> [w617]
                  shift-right: [w612] -> w558
                  shift-left: w562 -> [w615]
                  w613 = i32 ? ("ALG MSG queue")
                  n219 = local read "ALG output array"() -> (w611:T1)
                  n220 = call "VOC.vi"("input VOC ports"=w628, "voc states array"=w623, "output VOC ports"=w621, "Input VOC msg Array"=w620, "output VOC msg array"=w619, "ALG output array"=w611) -> ("Filled voc states array"=w622:cluster{u32, u8}[], "Modified input VOC ports"=w630:u8[], "Modified output VOC ports"=w629:u8[], "Clear Input VOC msg Array"=w618:T1, "output VOC array"=w616:T1)  [unwired: 5 in]
                  n221 = local write "Очередь сообщений для АУ"(w613) -> ()
                  n222 = local write "Очередь сообщений для  ВОУ"(w613) -> ()
                  n223 = call "CA.vi"("init input ports"=w629, "Alg states"=w625, "output"=w630, "input ALG msg array"=w617, "Output ALG msg array"=w615, "VOC output msg CASHE"=w616) -> ("Output Alg states"=w624:cluster{u32, u8}[], "input ports"=w626:u8[], "modified output ports"=w627:u8[], "Clear input msg Array"=w614:T1, "ALG output array"=w612:T1)  [unwired: 5 in]
                  "ALG output array" <- w612
                }
                "Result Input FOR VOC" <- w590
                "Array" <- w588
                n224 = call "PSConverter.vi"("Current States 2"=w587, "PROC"=w602, "STATES"=w599, "Input claster"=w584) -> ("Current States"=w585:string[][])
                n225 = property on="Отладочная информация процессов АУ" class="Tbl (strict)"("Value"=w585) -> ()  [unwired: 2 in, 2 out]
                n226 = call "PSConverter.vi"("Current States 2"=w581, "PROC"=w601, "STATES"=w600, "Input claster"=w582) -> ("Current States"=w580:string[][])
                n227 = local write "Отладочная информация процессов ВОУ"(w580) -> ()
                n228 = call "PortsArrayHandler.vi"("Input"=w590, "Init Input"=w591, "INPUT PORT states"=w593) -> ("Rezult Input Ports"=w556:u8[])  [unwired: 1 in]
                n229 = call "PortsArrayHandler.vi"("Input"=w588, "Init Input"=w589, "INPUT PORT states"=w594) -> ("Rezult Input Ports"=w557:u8[])  [unwired: 1 in]
                n230 = call "FormVarValuesArray.vi"("varables bytes"=w578, "varables ports"=w579, "Ports"=w557) -> ("Values Array"=w575:string[])  [unwired: 1 in]
                n231 = control-ref of="Входные порты ВОУ"() -> (w597:refnum<vi>)
                n232 = for {
                  tunnel: w597 -> [w605]
                  tunnel: u32 ? -> [w604]
                  tunnel: w556 -> [w603] mode=indexing
                  i -> [w606]
                  n233 = call "GUIUpdater.vi"("value"=w603, "Color"=w604, "line"=w606, "MCListbox Refnum"=w605) -> ()
                }
                n234 = local read "VOC Input varables bytes"() -> (w552:i32[])
                n235 = local read "VOC Input varables type"() -> (w545:string[])
                n236 = local read "VOC Input varables names"() -> (w544:string[])
                n237 = local read "VOC Input varables ports"() -> (w553:i32[])
                n238 = local read "AY Input varables names"() -> (w576:string[])
                n239 = local read "AY Input varables type"() -> (w577:string[])
                n240 = local read "VOC Output varables ports"() -> (w555:i32[])
                n241 = call "FormVarValuesArray.vi"("varables bytes"=w552, "varables ports"=w553, "Ports"=w556) -> ("Values Array"=w546:string[])  [unwired: 1 in]
                n242 = local read "VOC Output varables bytes"() -> (w554:i32[])
                n243 = call "FormVarValuesArray.vi"("varables bytes"=w571, "varables ports"=w572, "Ports"=w556) -> ("Values Array"=w568:string[])  [unwired: 1 in]
                n244 = local read "VOC Output varables type"() -> (w551:string[])
                n245 = Build Array(w545, w544, w546) -> (w547:string[][])
                n246 = local read "VOC Output varables names"() -> (w550:string[])
                n247 = local read "CA Output varables type"() -> (w567:string[])
                n248 = local read "CA Output varables names"() -> (w566:string[])
                n249 = call "FormVarValuesArray.vi"("varables bytes"=w554, "varables ports"=w555, "Ports"=w557) -> ("Values Array"=w549:string[])  [unwired: 1 in]
                n250 = Transpose 2D Array(2D array=w547) -> (transposed array=w543:string[][])
                n251 = control-ref of="ALG Input Ports"() -> (w598:refnum<vi>)
                n252 = for {
                  tunnel: w598 -> [w609]
                  tunnel: u32 ? -> [w608]
                  tunnel: w557 -> [w607] mode=indexing
                  i -> [w610]
                  n253 = call "GUIUpdater.vi"("value"=w607, "Color"=w608, "line"=w610, "MCListbox Refnum"=w609) -> ()
                }
                n254 = local write "Входные глобальные переменные ВОУ"(w543) -> ()
                n255 = Build Array(w577, w576, w575) -> (w574:string[][])
                n256 = Transpose 2D Array(2D array=w574) -> (transposed array=w573:string[][])
                n257 = local write "Входные глобальные переменные АУ"(w573) -> ()
                n258 = Build Array(w567, w566, w568) -> (w570:string[][])
                n259 = Build Array(w551, w550, w549) -> (w548:string[][])
                n260 = Transpose 2D Array(2D array=w570) -> (transposed array=w569:string[][])
                n261 = local write "Выходные глобальные переменные АУ"(w569) -> ()
                n262 = Transpose 2D Array(2D array=w548) -> (transposed array=w542:string[][])
                n263 = local write "Выходные глобальные переменные ВОУ"(w542) -> ()
              }
              frame #1 {
                n264 = local read "Curr step VOC MSG counter"() -> (w643:i32)
                n265 = control-ref of="Выходные сообщения от ВОУ на последнем шаге"() -> (w636:refnum<vi>)
                n266 = control-ref of="Список выходных сообщений от ВОУ"() -> (w637:refnum<vi>)
                n267 = control-ref of="Список выходных сообщений от АУ"() -> (w635:refnum<vi>)
                n268 = local read "Curr step ALG msg counter"() -> (w640:i32)
                n269 = control-ref of="Выходные сообщения от АУ на последнем шаге"() -> (w634:refnum<vi>)
                n270 = call "MsgParser.vi"("LAST MSGS"=w636, "MSG LOG"=w637, "MSG Counter"=w642, "current msg num"=w643) -> ("Result Counter"=w641:i32)  [unwired: 1 in]
                n271 = call "MsgParser.vi"("LAST MSGS"=w634, "MSG LOG"=w635, "MSG Counter"=w638, "current msg num"=w640) -> ("Result Counter"=w639:i32)  [unwired: 1 in]
              }
              frame #2 {
                n272 = call "LastStepMsgParser.vi"("Out MSG Names"=w647, "Out MSG Codes"=w646, "Msg Array"=w656) -> ("Output Alg Msg"=w655:string[][], "current msg num"=→"Curr step VOC MSG counter":i32)  [unwired: 5 in, 1 out]
                n273 = property on="Выходные сообщения от ВОУ на последнем шаге" class="MCListbox (strict)"("ItemNames"=w655) -> ()  [unwired: 2 in, 2 out]
                n274 = call "LastStepMsgParser.vi"("Out MSG Names"=w644, "Out MSG Codes"=w645, "Msg Array"=w651) -> ("Output Alg Msg"=w653:string[][], "current msg num"=→"Curr step ALG msg counter":i32)  [unwired: 5 in, 1 out]
                n275 = property on="Выходные сообщения от АУ на последнем шаге" class="MCListbox (strict)"("ItemNames"=w653) -> ()  [unwired: 2 in, 2 out]
                n276 = local read "Mode"() -> (w650:bool)
                n277 = local read "run"() -> (w649:bool)
                n278 = And(x=w650, y=w649) -> (x .and. y?=w648:bool)
                n279 = case shown="False" w648 {
                  frame #0 {
                    n280 = local write "stop 2"(bool ? ("stop 2")) -> ()
                    n281 = local write "run"(bool ? ("run")) -> ()
                  }
                  frame #1 {
                    n282 = local write "stop 2"(bool ? ("stop 2")) -> ()
                    n283 = local write "run"(bool ? ("run")) -> ()
                  }
                }
              }
            }
          }
        }
        n284 = call "FillMsgArray.vi"("Input VOC msg Array"=w278) -> ("Clear msg Array"=w265:T1)
        n285 = call "FillMsgArray.vi"("Input VOC msg Array"=w277) -> ("Clear msg Array"=w266:T1)
      }
    }
  }
